vi "Setup subWorkers.vi"(8 "error in":errorcluster, 11 "UserInterface in":refnum<class "UserInterface.lvclass">) -> (0 "error out":errorcluster, 3 "UserInterface out":refnum<class "UserInterface.lvclass">)   [LabVIEW 2021, in "UserInterface.lvclass"]
doc: "<b>Note: Do not change the code in this VI!</b>\nThis VI performs a setup of all the statically-linked subWorkers that belong to the Worker that calls this VI. This VI is created automatically by the 'Create/Add Worker' tool and must be called <b>before</b> any statically linked subWorkers are called."
uses:
  UserInterface.lvclass
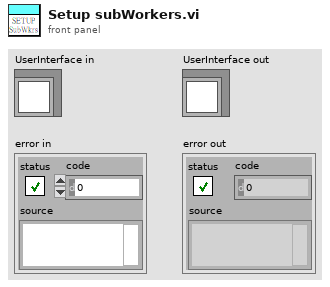
[diagram p1: front panel]
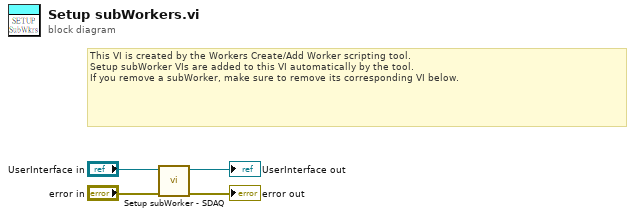
[diagram p0: block diagram]
diagram:
  # "This VI is created by the Workers Create/Add Worker scripting tool.\nSetup subWorker VIs are added to this VI automatically by the tool.\nIf you remove a subWorker, make sure to remove its corresponding VI below."
  n1 = call "Setup subWorker - SDAQ.vi"("error in"="error in", "UserInterface in"="UserInterface in") -> ("error out"=→"error out":errorcluster, "UserInterface out"=→"UserInterface out":refnum<class "UserInterface.lvclass">)  [unwired: 8 in]
